vi "LIDAR V4 FPGA Main.vi"() -> ()   [LabVIEW 2013]
uses:
  <vilib>/Platform/TimedLoop/XDataNode/timing_clust.ctl
  <vilib>/Platform/TimedLoop/XDataNode/nitl_modes.ctl
  <vilib>/Platform/TimedLoop/XDataNode/wakeup.ctl
  <vilib>/rvi/Emulation/niFpgaSctlEmulationGetInTimedLoop.vi
  <vilib>/rvi/Emulation/niFpgaEmulationReportErrorSimple.vi
  <vilib>/rvi/Emulation/niFpgaGetClockAttributes.vi
  <vilib>/rvi/Emulation/niFpgaCriticalErrorInLSC.vi
  <vilib>/rvi/FIFO/Fifo_Resource/nirvififoEmulationReadFpgaImpl.vi
  <vilib>/rvi/DataTransferAndStorage/Container/Common/niFpgaContainerGetUniqueNameForEmu.vi
  <vilib>/rvi/Memory/Memory_Emulation/nirvimemoryFastEmulationFpgaImpl.vi
  <instcachedir>/0/nirvimemoryFastEmulationFpgaImpl_5FBAB50466BC4C939F684F8805638BFC.lvgen/nirvimemoryFastEmulationFpgaImpl_5FBAB50466BC4C939F684F8805638BFC_016.vi
  <vilib>/rvi/Memory/Memory_Emulation/nirvimemoryFastEmulation.vi
  <vilib>/rvi/Memory/Memory_Emulation/nirvimemoryEmulation.vi
  <vilib>/rvi/eio/common/nirviEmuTemplateMethod_errors.vi
  <vilib>/rvi/FIFO/Fifo_Resource/nirvififoEmulationWriteFpgaImpl.vi
  <instcachedir>/0/nirvimemoryFastEmulationFpgaImpl_5FBAB50466BC4C939F684F8805638BFC.lvgen/nirvimemoryFastEmulationFpgaImpl_5FBAB50466BC4C939F684F8805638BFC_001.vi
  <vilib>/rvi/interface/RandomDataEmulation/nirviRandomDataFPGAFIFO.vi
  <vilib>/rvi/interface/RandomDataEmulation/niFpgaRandomDataHandleErrors.vi
  <vilib>/rvi/Emulation/niFpgaProcessEmulError.vi
  LIDAR V2 Globals.vi
  <vilib>/Platform/TimedLoop/XDataNode/XDataNode.xnode
  <vilib>/rvi/DataTransferAndStorage/Container/XNode/niFpgaContainer.xnode
  <vilib>/rvi/FIFO/Fifo_Resource/nirvififoEmulationRead.vi
  <vilib>/eio/EIONode/EIONode.xnode
  <vilib>/rvi/FIFO/Fifo_Resource/nirvififoEmulationWrite.vi
  <vilib>/rvi/interface/RandomDataEmulation/nirviRandomDataFpgaReadWriteTemplate.vi
  <vilib>/Platform/TimedLoop/XDataNode/XDNodeRunTimeDep.lvlib
panel:
  in  "ActiveLedIndexDeb":u16
  in  "LedScanDebEn":bool
  out "Port0":u8 format="%.0b"
  out "Port1Bit4":bool
  out "Port1Bit5":bool
  out "Port1":u8 format="%.0b"
  in  "FrameStartDisable":bool=TRUE
  in  "ScanMode":bool
  in  "ActiveLedIndex":u16
  in  "Start":bool
  in  "PattAdd":u32
  in  "PattData":u8
  in  "FillPatt":bool
  out "Timeouts":u16
  out "MemSel":bool
  out "LedIndex":u32
  in  "StreamToDMA":bool
  out "RawFifoWrite":bool
  in  "VgaAdd":u32
  in  "VgaData":i16
  in  "FillVga":bool
  in  "PFI2":bool
  in  "PFI3":bool
  in  "MaxStartSample":u32
  out "User Command Idle":bool
  out "User Command Status":u8
  out "User Error":bool
  out "Configured?":bool
  out "PLL Locked":bool
  in  "PulseIndex":i16
  in  "PulsePerLed":i16=199
  out "SimOut":i16
  out "EndOfPulseGen":bool
  in  "SampPerPattern":u32=100
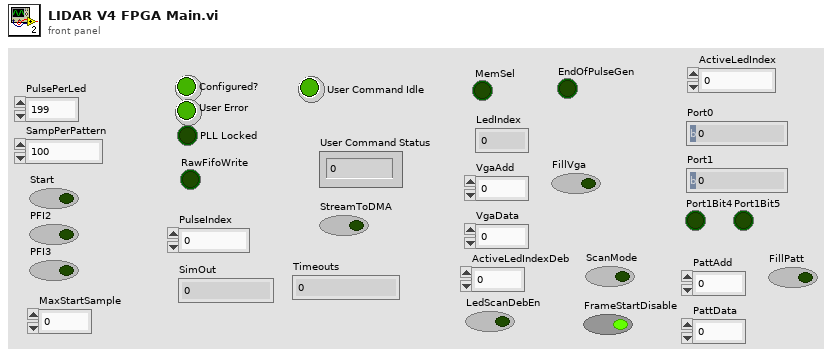
[diagram p1: front panel]
types:
  T1 = typedef "XDNodeRunTimeDep.lvlib/timing_clust.ctl" = cluster{"Expected End [f-1]":u64, "Actual End [f-1]":u64, "Finished Late? [f-1]":bool, "Expected End [i-1]":u64, "Actual End [i-1]":u64, "Finished Late? [i-1]":bool, "Expected Start [i]":u64, "Actual Start [i]":u64, "Expected Start [f]":u64, "Actual Start [f]":u64, "Source Name":string, "Structure Name":string, "Period":i64, "Deadline":i64, "Offset":i64, "Start":i64, "Priority":i32, "Timeout":i32, "Mode":T2, "Wakeup Reason":T3, "Error":errorcluster, "Source Type":string, "Secondary Source Type":string, "Global End Time":u64, "Global Start Time":u64, "Frame Duration":u64, "Iteration Duration":u64, "Assigned CPU":i32, "I/O Scan Engine Mode":u32}
  T2 = typedef "XDNodeRunTimeDep.lvlib/nitl_modes.ctl" = enum32{"No Change", "Process missed periods, maintain original phase", "Discard missed periods, maintain original phase", "Process missed periods, ignore original phase", "Discard missed periods, ignore original phase"}
  T3 = typedef "XDNodeRunTimeDep.lvlib/wakeup.ctl" = enum32{"Normal", "Aborted", "Asynchronous wakeup", "Timing source error", "Timed loop error", "Timeout"}
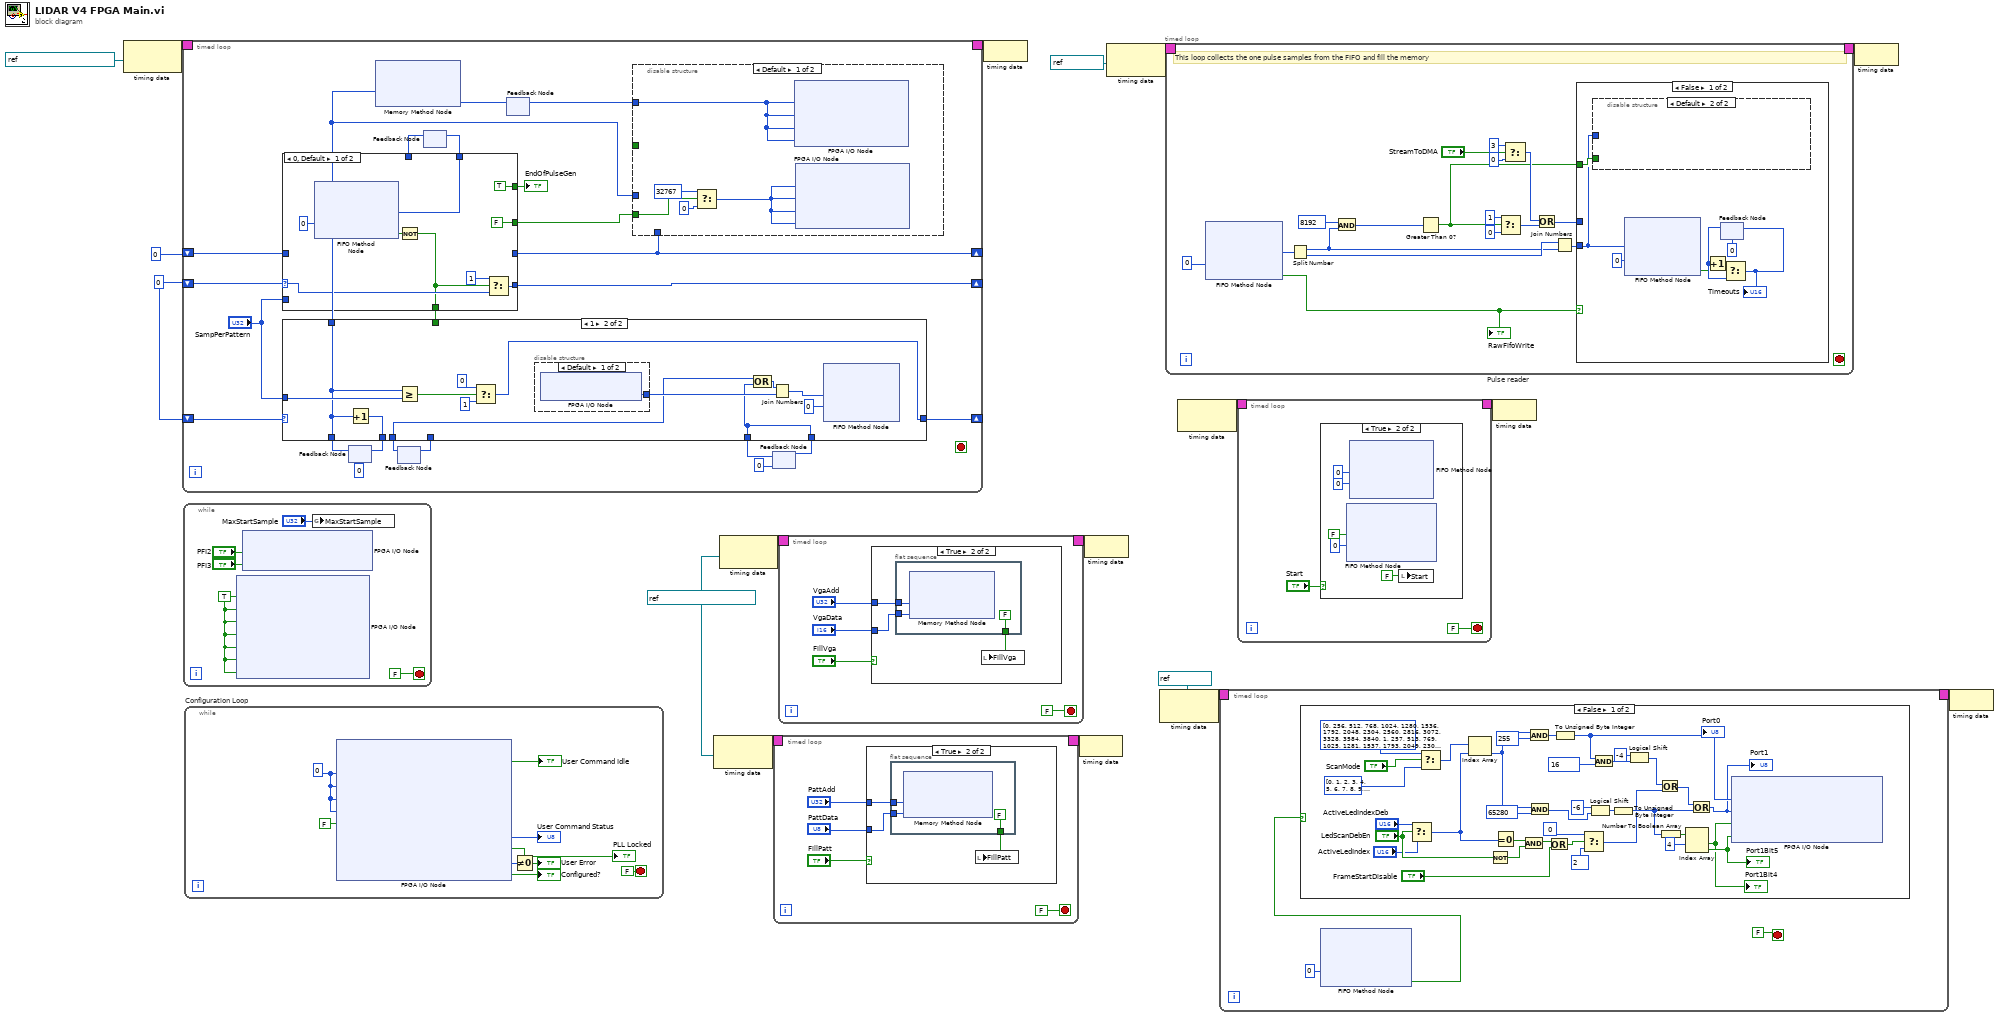
[diagram p0: block diagram]
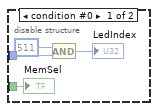
[diagram p5: hidden frame]
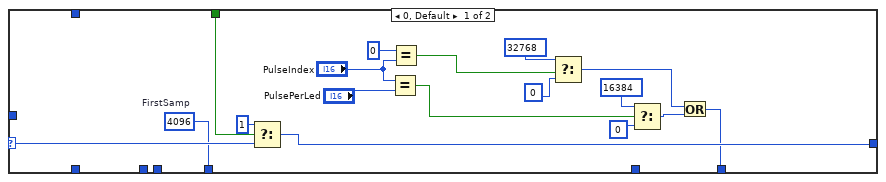
[diagram p8: hidden frame]
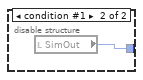
[diagram p9: hidden frame]
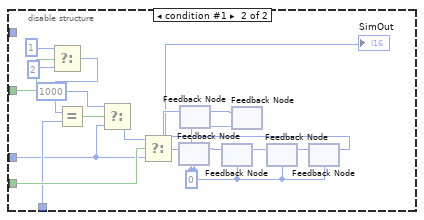
[diagram p10: hidden frame]
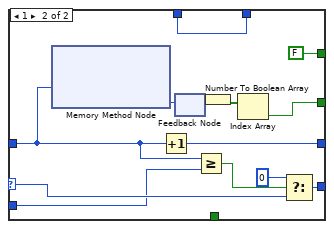
[diagram p11: hidden frame]
diagram:
  w4 = refnum<k21> "IO Module\\Data Clock" ("Source Name")
  w14 = u8 0
  n1 = node-c288(refnum<k21> "IO Module\\Data Clock" ("Source Name")) -> (w18:T1)
  n2 = timed-loop {
    timing: w18 -> [_]
    timing-out: [_] -> w17
    shift-right: [w40] -> _
    shift-left: w14 -> [w41]
    shift-right: [w38] -> _
    shift-left: u32 0 -> [w39]
    shift-right: [w33] -> _
    shift-left: w14 -> [w34]
    stop <- _ stop-if-true
    n3 = feedback #1(u32 0) -> (w23:u32)
    n4 = feedback #2() -> (w25:u16)  [unwired: 1 in]
    n5 = feedback #3() -> (w31:u16)  [unwired: 1 in]
    n6 = case shown="0, Default" w41 {
      selector: w41 -> [w99 w116]
      tunnel: [w104 w117] -> w40
      tunnel: w39 -> [_ w105]
      tunnel: [_ w110] -> w38
      tunnel: [FALSE w107] -> w37
      tunnel: "SampPerPattern" -> [_ w111]
      tunnel: [TRUE FALSE] -> w35
      tunnel: [w97 w112] -> w32
      tunnel: w31 -> [_ w112]
      tunnel: [w96 _] -> w19
      frame 0, Default {
        n7 = xnode ("FIFO Method Node")("Timeout"=0) -> ("Element"=w97:u16, "Timed Out?"=w102:bool)  [unwired: 1 in, 1 out]
        n8 = Not(x=w102) -> (.not. x?=w96:bool)
        n9 = Select(t=u8 1, s=w96, f=w99) -> (s? t:f=w104:u8)
      }
      frame 1 {
        n10 = xnode ("Memory Method Node")("Address"=w105) -> ("Data"=w109:u8)  [unwired: 1 in, 1 out]
        n11 = Increment(x=w105) -> (x+1=w110:u32)
        n12 = feedback-in #4(w109) -> ()
        n13 = feedback #4() -> (w106:u8)  [unwired: 1 in]
        n14 = Greater Or Equal?(x=w105, y=w111) -> (x >= y?=w114:bool)
        n15 = Number To Boolean Array(number=w106) -> (Boolean array=w108:bool[])
        n16 = Index Array(array=w108) -> (element=w107:bool)  [unwired: 1 in]
        n17 = Select(t=u8 0, s=w114, f=w116) -> (s? t:f=w117:u8)
      }
    }
    "EndOfPulseGen" <- w35
    n18 = feedback-in #3(w32) -> ()
    n19 = feedback #5() -> (w21:i16)  [unwired: 1 in]
    n20 = feedback #6(u16 0) -> (w27:u16)
    n21 = case shown="1" w34 {
      selector: w34 -> [w58 _]
      tunnel: [w56 w64] -> w33
      tunnel: w23 -> [_ w61]
      tunnel: [_ w71] -> w29
      tunnel: "SampPerPattern" -> [_ w70]
      tunnel: [w48 w63] -> w28
      tunnel: w27 -> [_ w63]
      tunnel: [w47 _] -> w26
      tunnel: w25 -> [_ w62]
      tunnel: [_ w61] -> w20
      tunnel: w19 -> [w44 _]
      frame 0, Default {
        w47 = u16 4096  # FirstSamp
        n22 = Select(t=u8 1, s=w44, f=w58) -> (s? t:f=w56:u8)
        n23 = Equal?(x="PulseIndex", y="PulsePerLed") -> (x = y?=w53:bool)
        n24 = Equal?(x=i16 0, y="PulseIndex") -> (x = y?=w51:bool)
        n25 = Select(t=u16 32768 ("FirstIterration"), s=w51, f=u16 0 ("x")) -> (s? t:f=w49:u16)
        n26 = Select(t=u16 16384 ("LastIterration"), s=w53, f=u16 0 ("x")) -> (s? t:f=w50:u16)
        n27 = Or(x=w49, y=w50) -> (x .or. y?=w48:u16)
      }
      frame 1 {
        n28 = Increment(x=w61) -> (x+1=w71:u32)
        n29 = Greater Or Equal?(x=w61, y=w70) -> (x >= y?=w69:bool)
        n30 = Select(t=u8 0, s=w69, f=u8 1) -> (s? t:f=w64:u8)
        n31 = disable-structure shown="Default" {
          disable-tunnel: [w72 w73] -> w65
          frame condition #0 (active) {
            n32 = xnode "FPGA I/O Node"() -> ("IO Module\\AI 0 N"=w72:i16)  [unwired: 1 in, 1 out]
          }
          frame condition #1 {
            n33 = local read "SimOut"() -> (w73:i16)
          }
        }
        n34 = Compound Arithmetic op=OR(w62, w63) -> (w66:u16)
        n35 = Join Numbers(hi=w66, lo=w65) -> ((hi.lo)=w60:u32)
        n36 = xnode ("FIFO Method Node")("Element"=w60, "Timeout"=0) -> ()  [unwired: 1 in, 2 out]
      }
    }
    n37 = feedback-in #1(w29) -> ()
    n38 = xnode ("Memory Method Node")("Address"=w20) -> ("Data"=w22:i16)  [unwired: 1 in, 1 out]
    n39 = feedback-in #2(w26) -> ()
    n40 = feedback-in #5(w22) -> ()
    n41 = disable-structure shown="Default" {
      disable-tunnel: w37 -> [w75 w89]
      disable-tunnel: w38 -> [_ w88]
      disable-tunnel: w21 -> [w74 _]
      disable-tunnel: w20 -> [_ w84]
      disable-tunnel: _ -> [_ w79]
      frame condition #0 (active) {
        n42 = Select(t=i16 32767 ("IO Module\\AO 0 N"), s=w75, f=i16 0) -> (s? t:f=w76:i16)
        n43 = xnode "FPGA I/O Node"("IO Module\\AO 1 N"=w74, "IO Module\\AO 1 N-1"=w74, "IO Module\\AO 1 N-2"=w74, "IO Module\\AO 1 N-3"=w74) -> ()  [unwired: 4 in, 4 out]
        n44 = xnode "FPGA I/O Node"("IO Module\\AO 0 N-3"=w76, "IO Module\\AO 0 N-2"=w76, "IO Module\\AO 0 N-1"=w76, "IO Module\\AO 0 N"=w76) -> ()  [unwired: 4 in, 4 out]
      }
      frame condition #1 {
        w90 = i16 0 ("IO Module\\AO 0")
        n45 = Select(t=u16 1 ("x"), s=w79, f=u16 2 ("x")) -> (s? t:f=w80:u16)
        n46 = Equal?(x=w80, y=w88) -> (x = y?=w86:bool)
        n47 = Select(t=i16 1000 ("IO Module\\AO 0"), s=w86, f=w84) -> (s? t:f=w87:u32)
        n48 = Select(t=w87, s=w89, f=w84) -> (s? t:f=w83:u32)
        "SimOut" <- w83
        n49 = feedback-in #7(w83) -> ()
        n50 = feedback #7(w90) -> (w95:u32)
        n51 = feedback #8(w90) -> (w91:u32)
        n52 = feedback #9(w90) -> (w94:u32)
        n53 = feedback-in #9(w95) -> ()
        n54 = feedback #10(w90) -> ()  [unwired: 1 in]
        n55 = feedback-in #10(w91) -> ()
        n56 = feedback #11(w90) -> (w93:u32)
        n57 = feedback-in #11(w94) -> ()
        n58 = feedback #12(w90) -> (w92:u32)
        n59 = feedback-in #8(w92) -> ()
        n60 = feedback-in #12(w93) -> ()
      }
    }
    n61 = feedback-in #6(w28) -> ()
  }
  n62 = while {
    stop <- FALSE stop-if-true
    w123 = TRUE ("IO Module\\DIO Port 0 WE")
    n63 = xnode "FPGA I/O Node"("IO Module\\DIO Port 0 WE"=w123, "IO Module\\DIO Port 1 WE"=w123, "IO Module\\PFI 0 WE"=w123, "IO Module\\PFI 1 WE"=w123, "IO Module\\PFI 2 WE"=w123, "IO Module\\PFI 3 WE"=w123, "IO Module\\AO Data Sync"=w123) -> ()  [unwired: 7 in, 7 out]
    n64 = xnode "FPGA I/O Node"("IO Module\\PFI 2 Wr Data"="PFI2", "IO Module\\PFI 3 Wr Data"="PFI3") -> ()  [unwired: 2 in, 2 out]
    n65 = global write "LIDAR V2 Globals.vi" "MaxStartSample"("MaxStartSample") -> ()
  }
  n66 = while "Configuration Loop" {
    stop <- FALSE stop-if-true
    w126 = u8 0 ("SPI Device")
    n67 = xnode "FPGA I/O Node"("IO Module\\SPI Device"=w126, "IO Module\\User Command"=w126, "IO Module\\User Data 0"=w126, "IO Module\\User Data 1"=w126, "IO Module\\User Command Commit"=FALSE ("IO Module\\User Command Commit")) -> ("IO Module\\User Command Idle"=→"User Command Idle":bool, "IO Module\\User Command Status"=→"User Command Status":u8, "IO Module\\PLL Locked"=→"PLL Locked":bool, "IO Module\\User Error"=w130:u8, "IO Module\\Initialization Done"=→"Configured?":bool)  [unwired: 10 in, 10 out]
    n68 = Not Equal To 0?(x=w130) -> (x != 0?=→"User Error":bool)
  }
  n69 = node-c288(w4) -> (w8:T1)
  n70 = node-c288(w4) -> (w13:T1)
  n71 = timed-loop {
    timing: w8 -> [_]
    timing-out: [_] -> w7
    stop <- FALSE stop-if-true
    n72 = case shown="True" "FillPatt" {
      tunnel: "PattAdd" -> [_ w140]
      tunnel: "PattData" -> [_ w139]
      frame False {
      }
      frame True {
        n73 = flat-sequence {
          tunnel: w140 -> [w143]
          tunnel: w139 -> [w142]
          tunnel: [FALSE ("FillVga")] -> w138
          frame #0 {
            n74 = xnode ("Memory Method Node")("Address"=w143, "Data"=w142) -> ()  [unwired: 1 in, 1 out]
          }
        }
        n75 = local write "FillPatt"(w138) -> ()
      }
    }
  }
  n76 = timed-loop {
    timing: w13 -> [_]
    timing-out: [_] -> w12
    stop <- FALSE stop-if-true
    n77 = case shown="True" "FillVga" {
      tunnel: "VgaAdd" -> [_ w152]
      tunnel: "VgaData" -> [_ w151]
      frame False {
      }
      frame True {
        n78 = flat-sequence {
          tunnel: w152 -> [w155]
          tunnel: w151 -> [w154]
          tunnel: [FALSE ("FillVga")] -> w150
          frame #0 {
            n79 = xnode ("Memory Method Node")("Address"=w155, "Data"=w154) -> ()  [unwired: 1 in, 1 out]
          }
        }
        n80 = local write "FillVga"(w150) -> ()
      }
    }
  }
  n81 = node-c288(w17) -> ()
  n82 = node-c288(w7) -> ()
  n83 = node-c288(w12) -> ()
  n84 = node-c288(refnum<k21> "130MHz" ("Source Name")) -> (w11:T1)
  n85 = node-c288(refnum<k21> "130MHz" ("Source Name")) -> (w3:T1)
  n86 = timed-loop "Pulse reader" {
    timing: w11 -> [_]
    timing-out: [_] -> w10
    stop <- _ stop-if-true
    # "This loop collects the one pulse samples from the FIFO and fill the memory"
    n87 = xnode ("FIFO Method Node")("Timeout"=0) -> ("Element"=w160:u32, "Timed Out?"=w158:bool)  [unwired: 1 in, 1 out]
    "RawFifoWrite" <- w158
    n88 = Split Number(x=w160) -> (hi(x)=w161:u16, lo(x)=w164:u16)
    n89 = And(x=u16 8192, y=w161) -> (x .and. y?=w167:u16)
    n90 = Greater Than 0?(x=w167) -> (x > 0?=w162:bool)
    n91 = Select(t=i16 1, s=w162, f=i16 0) -> (s? t:f=w171:i16)
    n92 = Select(t=i16 3, s="StreamToDMA", f=i16 0) -> (s? t:f=w170:i16)
    n93 = Or(x=w170, y=w171) -> (x .or. y?=w166:i16)
    n94 = Join Numbers(hi=w164, lo=w161) -> ((hi.lo)=w163:u32)
    n95 = case shown="False" w158 {
      tunnel: w166 -> [_ _]
      tunnel: w163 -> [w181 _]
      tunnel: w162 -> [w182 _]
      frame False {
        n96 = disable-structure shown="Default" {
          disable-tunnel: w182 -> [w186 _]
          disable-tunnel: w181 -> [w185 _]
          frame condition #0 {
            n97 = And(x=u32 511, y=w185) -> (x .and. y?=→"LedIndex":u32)
            "MemSel" <- w186
          }
          frame condition #1 (active) {
          }
        }
        n98 = xnode ("FIFO Method Node")("Element"=w181, "Timeout"=0) -> ("Timed Out?"=w176:bool)  [unwired: 1 in, 1 out]
        n99 = feedback #13(u16 0) -> (w179:u16)
        n100 = Increment(x=w179) -> (x+1=w180:u16)
        n101 = Select(t=w180, s=w176, f=w179) -> (s? t:f=w178:u16)
        "Timeouts" <- w178
        n102 = feedback-in #13(w178) -> ()
      }
      frame True {
      }
    }
  }
  n103 = node-c288() -> (w6:T1)  [unwired: 1 in]
  n104 = timed-loop {
    timing: w3 -> [_]
    timing-out: [_] -> w2
    stop <- FALSE stop-if-true
    n105 = xnode ("FIFO Method Node")("Timeout"=0) -> ("Timed Out?"=w189:bool)  [unwired: 1 in, 2 out]
    n106 = case shown="False" w189 {
      frame False {
        n107 = Select(t="ActiveLedIndexDeb", s="LedScanDebEn", f="ActiveLedIndex") -> (s? t:f=w208:u16)
        n108 = Select(t=u16[] [0, 256, 512, 768, 1024, 1280, 1536, 1792, 2048, 2304, 2560, 2816, 3072, 3328, 3584, 3840, 1, 257, 513, 769, 1025, 1281, 1537, 1793, 2049, 2305, 2561, 2817, 3073, 3329, 3585, 3841, 2, 258, 514, 770, 1026, 1282, 1538, 1794, 2050, 2306, 2562, 2818, 3074, 3330, 3586, 3842, 3, 259, 515, 771, 1027, 1283, 1539, 1795, 2051, 2307, 2563, 2819, 3075, 3331, 3587, 3843, 4, 260, 516, 772, 1028, 1284, 1540, 1796, 2052, 2308, 2564, 2820, 3076, 3332, 3588, 3844, 5, 261, 517, 773, 1029, 1285, 1541, 1797, 2053, 2309, 2565, 2821, 3077, 3333, 3589, 3845, 6, 262, 518, 774, 1030, 1286, 1542, 1798, 2054, 2310, 2566, 2822, 3078, 3334, 3590, 3846, 7, 263, 519, 775, 1031, 1287, 1543, 1799, 2055, 2311, 2567, 2823, 3079, 3335, 3591, 3847, 8, 264, 520, 776, 1032, 1288, 1544, 1800, 2056, 2312, 2568, 2824, 3080, 3336, 3592, 3848, 9, 265, 521, 777, 1033, 1289, 1545, 1801, 2057, 2313, 2569, 2825, 3081, 3337, 3593, 3849, 10, 266, 522, 778, 1034, 1290, 1546, 1802, 2058, 2314, 2570, 2826, 3082, 3338, 3594, 3850, 11, 267, 523, 779, 1035, 1291, 1547, 1803, 2059, 2315, 2571, 2827, 3083, 3339, 3595, 3851, 12, 268, 524, 780, 1036, 1292, 1548, 1804, 2060, 2316, 2572, 2828, 3084, 3340, 3596, 3852, 13, 269, 525, 781, 1037, 1293, 1549, 1805, 2061, 2317, 2573, 2829, 3085, 3341, 3597, 3853, 14, 270, 526, 782, 1038, 1294, 1550, 1806, 2062, 2318, 2574, 2830, 3086, 3342, 3598, 3854, 15, 271, 527, 783, 1039, 1295, 1551, 1807, 2063, 2319, 2575, 2831, 3087, 3343, 3599, 3855, 16, 272, 528, 784, 1040, 1296, 1552, 1808, 2064, 2320, 2576, 2832, 3088, 3344, 3600, 3856, 17, 273, 529, 785, 1041, 1297, 1553, 1809, 2065, 2321, 2577, 2833, 3089, 3345, 3601, 3857, 18, 274, 530, 786, 1042, 1298, 1554, 1810, 2066, 2322, 2578, 2834, 3090, 3346, 3602, 3858, 19, 275, 531, 787, 1043, 1299, 1555, 1811, 2067, 2323, 2579, 2835, 3091, 3347, 3603, 3859] ("Array"), s="ScanMode", f=u16[] [0, 1, 2, 3, 4, 5, 6, 7, 8, 9, 10, 11, 12, 13, 14, 15, 16, 17, 18, 19, 256, 257, 258, 259, 260, 261, 262, 263, 264, 265, 266, 267, 268, 269, 270, 271, 272, 273, 274, 275, 512, 513, 514, 515, 516, 517, 518, 519, 520, 521, 522, 523, 524, 525, 526, 527, 528, 529, 530, 531, 768, 769, 770, 771, 772, 773, 774, 775, 776, 777, 778, 779, 780, 781, 782, 783, 784, 785, 786, 787, 1024, 1025, 1026, 1027, 1028, 1029, 1030, 1031, 1032, 1033, 1034, 1035, 1036, 1037, 1038, 1039, 1040, 1041, 1042, 1043, 1280, 1281, 1282, 1283, 1284, 1285, 1286, 1287, 1288, 1289, 1290, 1291, 1292, 1293, 1294, 1295, 1296, 1297, 1298, 1299, 1536, 1537, 1538, 1539, 1540, 1541, 1542, 1543, 1544, 1545, 1546, 1547, 1548, 1549, 1550, 1551, 1552, 1553, 1554, 1555, 1792, 1793, 1794, 1795, 1796, 1797, 1798, 1799, 1800, 1801, 1802, 1803, 1804, 1805, 1806, 1807, 1808, 1809, 1810, 1811, 2048, 2049, 2050, 2051, 2052, 2053, 2054, 2055, 2056, 2057, 2058, 2059, 2060, 2061, 2062, 2063, 2064, 2065, 2066, 2067, 2304, 2305, 2306, 2307, 2308, 2309, 2310, 2311, 2312, 2313, 2314, 2315, 2316, 2317, 2318, 2319, 2320, 2321, 2322, 2323, 2560, 2561, 2562, 2563, 2564, 2565, 2566, 2567, 2568, 2569, 2570, 2571, 2572, 2573, 2574, 2575, 2576, 2577, 2578, 2579, 2816, 2817, 2818, 2819, 2820, 2821, 2822, 2823, 2824, 2825, 2826, 2827, 2828, 2829, 2830, 2831, 2832, 2833, 2834, 2835, 3072, 3073, 3074, 3075, 3076, 3077, 3078, 3079, 3080, 3081, 3082, 3083, 3084, 3085, 3086, 3087, 3088, 3089, 3090, 3091, 3328, 3329, 3330, 3331, 3332, 3333, 3334, 3335, 3336, 3337, 3338, 3339, 3340, 3341, 3342, 3343, 3344, 3345, 3346, 3347, 3584, 3585, 3586, 3587, 3588, 3589, 3590, 3591, 3592, 3593, 3594, 3595, 3596, 3597, 3598, 3599, 3600, 3601, 3602, 3603, 3840, 3841, 3842, 3843, 3844, 3845, 3846, 3847, 3848, 3849, 3850, 3851, 3852, 3853, 3854, 3855, 3856, 3857, 3858, 3859] ("Array")) -> (s? t:f=w194:u16[])
        n109 = Index Array(array=w194, index=w208) -> (element=w220:u16)
        n110 = Not(x="LedScanDebEn") -> (.not. x?=w205:bool)
        n111 = Equal To 0?(x=w208) -> (x = 0?=w207:bool)
        n112 = And(x=w207, y=w205) -> (x .and. y?=w203:bool)
        n113 = And(x=w220, y=u16 255) -> (x .and. y?=w218:u16)
        n114 = And(x=w220, y=u16 65280) -> (x .and. y?=w217:u16)
        n115 = Or(x=w203, y="FrameStartDisable") -> (x .or. y?=w198:bool)
        n116 = To Unsigned Byte Integer(number=w218) -> (unsigned 8bit integer=w214:u8)
        "Port0" <- w214
        n117 = Select(t=u8 0, s=w198, f=u8 2) -> (s? t:f=w200:u8)
        n118 = Logical Shift(y=i16 -6, x=w217) -> (x << y=w216:u16)
        n119 = And(x=w214, y=u8 16) -> (x .and. y?=w213:u8)
        n120 = To Unsigned Byte Integer(number=w216) -> (unsigned 8bit integer=w210:u8)
        n121 = Logical Shift(y=i16 -4, x=w213) -> (x << y=w204:u8)
        n122 = Or(x=w204, y=w200) -> (x .or. y?=w199:u8)
        n123 = Number To Boolean Array(number=w210) -> (Boolean array=w226:bool[])
        n124 = Index Array(array=w226, index #1=4 ("index")) -> (element #1=w211:bool, element #2=w224:bool)  [unwired: 1 in]
        "Port1Bit4" <- w211
        "Port1Bit5" <- w224
        n125 = Or(x=w199, y=w210) -> (x .or. y?=w209:u8)
        "Port1" <- w209
        n126 = xnode "FPGA I/O Node"("IO Module\\DIO Port 0 Wr Data"=w214, "IO Module\\DIO Port 1 Wr Data"=w209, "IO Module\\PFI 0 Wr Data"=w211, "IO Module\\PFI 1 Wr Data"=w224) -> ()  [unwired: 4 in, 4 out]
      }
      frame True {
      }
    }
  }
  n127 = timed-loop {
    timing: w6 -> [_]
    timing-out: [_] -> w5
    stop <- FALSE stop-if-true
    n128 = case shown="True" "Start" {
      frame False {
      }
      frame True {
        n129 = xnode ("FIFO Method Node")("Element"=FALSE, "Timeout"=0) -> ()  [unwired: 1 in, 2 out]
        n130 = xnode ("FIFO Method Node")("Element"=u16 0, "Timeout"=0) -> ()  [unwired: 1 in, 2 out]
        n131 = local write "Start"(FALSE ("Start")) -> ()
      }
    }
  }
  n132 = node-c288(w5) -> ()
  n133 = node-c288(w10) -> ()
  n134 = node-c288(w2) -> ()
